vi "Complementary Angle (scalar).vi"(7 "angle units":T1 items=["radian in, radian out", "radian in, degree out", "degree in, degree out", "degree in, radian out"], 11 "angle":dbl) -> (0 "error":i32, 3 "complementary angle":dbl)   [LabVIEW 2020, in "NI_AAL_Angle.lvlib"]
doc: "Calculates the complementary angle of the input angle.\n\nWire data to any of the angle inputs to determine the polymorphic instance to use or manually select the instance."
uses:
  <vilib>/Analysis/NI_AAL_Angle.lvlib
  <vilib>/Analysis/coordinate.llb/Angle Units.ctl
  <vilib>/Analysis/coordinate.llb/Angle Range (Degree).ctl
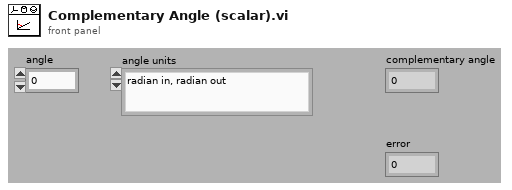
[diagram p1: front panel]
types:
  T1 = typedef "NI_AAL_Angle.lvlib/Angle Units.ctl" = i32
  T2 = typedef "NI_AAL_Angle.lvlib/Angle Range (Degree).ctl" = u16
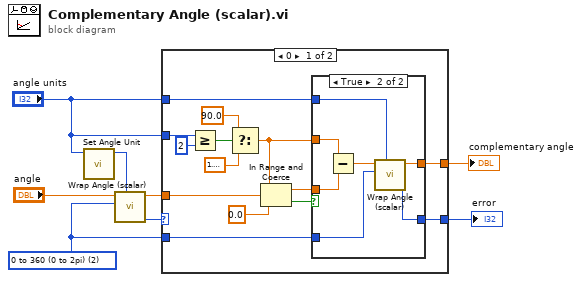
[diagram p0: block diagram]
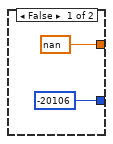
[diagram p2: hidden frame]
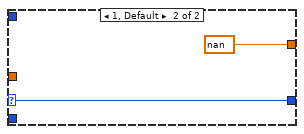
[diagram p3: hidden frame]
diagram:
  w1 = T2 2 items=["none", "-180 to 180 (-pi to pi)", "0 to 360 (0 to 2pi)"] ("angle range")
  n1 = call <vilib>:"Set Angle Unit.vi"("angle units in"="angle units") -> ("angle units out"=w5:T1)  [unwired: 10 in]
  n2 = call <vilib>:"Wrap Angle (scalar).vi"("angle units"=w5, "angle range"=w1, "angle in"="angle") -> ("error"=w7:i32, "angle out"=w6:dbl)  [unwired: 7 in]
  n3 = case shown="0" w7 {
    selector: w7 -> [_ w32]
    tunnel: w6 -> [w22 _]
    tunnel: "angle units" -> [w21 _]
    tunnel: [w12 nan] -> w4
    tunnel: [w11 w32] -> w3
    tunnel: "angle units" -> [w10 _]
    tunnel: w1 -> [w9 _]
    frame 0 {
      n4 = Greater Or Equal?(x=w21, y=2) -> (x >= y?=w18:bool)
      n5 = Select(t=90.0, s=w18, f=1.5707963267948966) -> (s? t:f=w13:dbl)
      n6 = In Range and Coerce(upper limit=w13, x=w22, lower limit=0.0 ("upper limit")) -> (coerced(x)=w14:dbl, In Range?=w15:bool)
      n7 = case shown="True" w15 {
        tunnel: w14 -> [_ w31]
        tunnel: w13 -> [_ w30]
        tunnel: [nan w28] -> w12
        tunnel: [-20106 w25] -> w11
        tunnel: w10 -> [_ w27]
        tunnel: w9 -> [_ w26]
        frame False {
        }
        frame True {
          n8 = Subtract(x=w30, y=w31) -> (x-y=w29:dbl)
          n9 = call <vilib>:"Wrap Angle (scalar).vi"("angle units"=w27, "angle range"=w26, "angle in"=w29) -> ("error"=w25:i32, "angle out"=w28:dbl)  [unwired: 7 in]
        }
      }
    }
    frame 1, Default {
    }
  }
  "complementary angle" <- w4
  "error" <- w3
